vi "DriverStationSendData.vi"   [LabVIEW 2023]
doc: "This VI continously sends data from the robot to the FRC 4265 Dashboard, the joysticks, and the FIRST Driver Station. Data are only sent to the network tables when values change. Detailed sensor data are only sent when the user is currently viewing the Tune tab on the FRC 4265 Dashboard."
uses:
  <vilib>/Rock Robotics/WPI/DriverStation/WPI_DriverStationAllianceInfo.ctl
  0776bb0e-5b58-4af6-957d-bc8a00d122f2.vi
  c0b3d222-824d-4eea-b194-4551ccfede72.vi
  8db4f2bd-6a8b-4c46-90ec-c7212a8cd13c.vi
  7bef9c9e-0ebd-49c4-875e-b1a7c8331b9c.vi
  25034f12-7a14-4040-b0c6-1082a0a618fc.vi
  de71cbf9-497c-4b6e-9325-f91bd1a1ea26.vi
  fe406e7d-1768-469c-a538-67ef48fe7f0a.vi
  b740731d-63e7-4115-93ae-b3fbc4be728c.vi
  770be32f-1451-480f-be59-c95d907125ff.vi
  9b798e4d-9237-4864-9935-e997a6382231.vi
  bf36f1cc-a3b1-4189-9382-aff2debcdd91.vi
  09cab74e-98ba-4de8-92cd-b77291f0cae9.vi
  e0f98f21-d526-4ef5-b75c-6f3c78a33603.vi
  36759aca-d9c6-44a3-918a-9a0e895c718f.vi
  d2dc3f3f-39b5-4c17-a933-05bbedc8d5d9.vi
  47e8091e-0604-4560-b6ee-932fcc40f94c.vi
  040c557e-2b24-4d13-8fef-d98c711cf45f.vi
  89115614-314f-44eb-b4c5-fafba5d31cd4.vi
  9f98788f-6f1b-4a83-a100-7d872b9f460c.vi
  d5b4d43d-cd94-4278-ad04-5030dc28ac17.vi
  c90139ce-4630-4044-962b-b9323bb651b8.vi
  85014151-be37-4cbe-9458-644b8a18b20e.vi
  8274615e-b3b9-4435-b2de-484384c0ad12.vi
  e1fb6d49-71d8-4856-b92a-968cf29c63e6.vi
  9baabde0-90b0-49bc-8c7c-ecb50ab3c219.vi
  7c9ec5b3-0cab-420b-b9c6-0eeed636b797.vi
  a8a67854-f7a1-4059-85f2-a1af3b07aa69.vi
  f0e3ca73-5587-4f60-abb3-83c549356a0b.vi
  135be689-108c-4a89-9837-55c31bad5bbe.vi
  90b8ffb3-02b0-4f37-8578-c415475fcf1f.vi
  26471c2c-aca7-4047-a7cd-e40da11d04c1.vi
  0c9c2ce5-4f8f-4d2f-a61f-dde9fdddd21a.vi
  948ebb5e-1fee-45f5-b788-843df8d92f11.vi
  07cec073-88f4-4f05-94a3-d05e12405c4e.vi
  c10cd8a7-bdb7-4c92-ac5c-00af4ab7dc85.vi
  ce82ba1c-dcc2-498f-8d23-146b12230de2.vi
  cbbdf295-aa1d-4db8-8566-cac5820e4458.vi
  52d993e2-6fbc-4ee4-b085-b3f80a4c3067.vi
  5ccc8aa6-325d-4660-b060-52e30b1d582a.vi
  296afef1-bc02-48ee-92b6-09523bb21575.vi
  811948b9-57e2-4f47-a6f6-f2932d14082f.vi
  5739ca73-a30d-4c92-9c50-72d6edc45fc4.vi
  0620df73-5841-450f-a219-dd10bb38cbc0.vi
  fb087c59-fbb1-4979-ba7d-d29f083bcd8a.vi
  94826c24-d30e-4eee-b4d4-6d626a9b9fe7.vi
  fa7611ee-6daf-4341-84ec-bae2216748b8.vi
  75656f7d-003f-4895-8150-fd75ccee7ba7.vi
  2a5192f0-5560-467f-8dc7-b3093601f5e6.vi
  41cc3bc6-bbb3-49f6-8be0-59cefde1612f.vi
  f5eb47e9-f0d5-4358-ba2d-5c1ea061b043.vi
  7ab91d4b-7be3-4017-93bd-af9165b60b99.vi
  f2a1d575-33e9-46b9-ab25-b575ffc27caf.vi
  2130d5a6-5db2-43ac-bd1b-a97f99664b9f.vi
  375a6e8a-27f7-4291-b992-01fa32110d43.vi
  cffa72e0-3c7a-4932-a37a-7040beb2a623.vi
  ec159192-b170-40c4-82c6-c3d920d678b2.vi
  f6387c7a-a3bd-4a9d-91dd-fe2f33c833ae.vi
  03661406-2ba7-4cad-bba1-149348653281.vi
  d97fc881-b6e7-47be-8bf3-d72bdee58bbc.vi
  29b9fc74-ab20-4616-a405-8bf0304d7e4e.vi
  d8771982-752a-4faa-9266-2bef2163cf3a.vi
  7b6a1411-5027-49fa-871d-ec9f81e31f95.vi
  20dd8ad3-6bbc-4cac-b559-7f798e2b6680.vi
  5e95d400-1295-40c5-af46-ec5444c3a2ff.vi
  d5b53c9f-0752-48c4-83e9-94c6e20357af.vi
  a2a431f6-075f-4920-bddd-4a0a2690fbc3.vi
  63edfc8b-2713-4fb9-bbf0-712b13f7ed91.vi
  5dc304d7-e71b-4cd2-8d9d-954937278b50.vi
  e1c3efee-a4b9-4741-b362-77d4d14dba05.vi
  c227876e-c49d-4561-a8c1-0ac62d9f5df0.vi
  e617f737-58a4-4889-9924-01a8da667f92.vi
  a9076398-35a2-42a7-b542-3dd64d126b59.vi
  44842b00-b9c8-4b1f-a6e0-fc22f00ef89a.vi
  8db4f2bd-6a8b-4c46-90ec-c7212a8cd13c.vi/77c742ae-e671-49bb-a825-a6e8cebc9f63.vi
  7bef9c9e-0ebd-49c4-875e-b1a7c8331b9c.vi/77c742ae-e671-49bb-a825-a6e8cebc9f63.vi
  25034f12-7a14-4040-b0c6-1082a0a618fc.vi/77c742ae-e671-49bb-a825-a6e8cebc9f63.vi
  de71cbf9-497c-4b6e-9325-f91bd1a1ea26.vi/77c742ae-e671-49bb-a825-a6e8cebc9f63.vi
  fe406e7d-1768-469c-a538-67ef48fe7f0a.vi/77c742ae-e671-49bb-a825-a6e8cebc9f63.vi
  b740731d-63e7-4115-93ae-b3fbc4be728c.vi/77c742ae-e671-49bb-a825-a6e8cebc9f63.vi
  770be32f-1451-480f-be59-c95d907125ff.vi/77c742ae-e671-49bb-a825-a6e8cebc9f63.vi
  9b798e4d-9237-4864-9935-e997a6382231.vi/77c742ae-e671-49bb-a825-a6e8cebc9f63.vi
  bf36f1cc-a3b1-4189-9382-aff2debcdd91.vi/77c742ae-e671-49bb-a825-a6e8cebc9f63.vi
  09cab74e-98ba-4de8-92cd-b77291f0cae9.vi/77c742ae-e671-49bb-a825-a6e8cebc9f63.vi
  e0f98f21-d526-4ef5-b75c-6f3c78a33603.vi/77c742ae-e671-49bb-a825-a6e8cebc9f63.vi
  36759aca-d9c6-44a3-918a-9a0e895c718f.vi/77c742ae-e671-49bb-a825-a6e8cebc9f63.vi
  d2dc3f3f-39b5-4c17-a933-05bbedc8d5d9.vi/77c742ae-e671-49bb-a825-a6e8cebc9f63.vi
  47e8091e-0604-4560-b6ee-932fcc40f94c.vi/77c742ae-e671-49bb-a825-a6e8cebc9f63.vi
  040c557e-2b24-4d13-8fef-d98c711cf45f.vi/77c742ae-e671-49bb-a825-a6e8cebc9f63.vi
  89115614-314f-44eb-b4c5-fafba5d31cd4.vi/77c742ae-e671-49bb-a825-a6e8cebc9f63.vi
  9f98788f-6f1b-4a83-a100-7d872b9f460c.vi/77c742ae-e671-49bb-a825-a6e8cebc9f63.vi
  d5b4d43d-cd94-4278-ad04-5030dc28ac17.vi/77c742ae-e671-49bb-a825-a6e8cebc9f63.vi
  c90139ce-4630-4044-962b-b9323bb651b8.vi/77c742ae-e671-49bb-a825-a6e8cebc9f63.vi
  85014151-be37-4cbe-9458-644b8a18b20e.vi/77c742ae-e671-49bb-a825-a6e8cebc9f63.vi
  8274615e-b3b9-4435-b2de-484384c0ad12.vi/77c742ae-e671-49bb-a825-a6e8cebc9f63.vi
  e1fb6d49-71d8-4856-b92a-968cf29c63e6.vi/77c742ae-e671-49bb-a825-a6e8cebc9f63.vi
  9baabde0-90b0-49bc-8c7c-ecb50ab3c219.vi/77c742ae-e671-49bb-a825-a6e8cebc9f63.vi
  7c9ec5b3-0cab-420b-b9c6-0eeed636b797.vi/77c742ae-e671-49bb-a825-a6e8cebc9f63.vi
  a8a67854-f7a1-4059-85f2-a1af3b07aa69.vi/77c742ae-e671-49bb-a825-a6e8cebc9f63.vi
  f0e3ca73-5587-4f60-abb3-83c549356a0b.vi/77c742ae-e671-49bb-a825-a6e8cebc9f63.vi
  135be689-108c-4a89-9837-55c31bad5bbe.vi/77c742ae-e671-49bb-a825-a6e8cebc9f63.vi
  90b8ffb3-02b0-4f37-8578-c415475fcf1f.vi/77c742ae-e671-49bb-a825-a6e8cebc9f63.vi
  26471c2c-aca7-4047-a7cd-e40da11d04c1.vi/77c742ae-e671-49bb-a825-a6e8cebc9f63.vi
  0c9c2ce5-4f8f-4d2f-a61f-dde9fdddd21a.vi/77c742ae-e671-49bb-a825-a6e8cebc9f63.vi
  948ebb5e-1fee-45f5-b788-843df8d92f11.vi/77c742ae-e671-49bb-a825-a6e8cebc9f63.vi
  07cec073-88f4-4f05-94a3-d05e12405c4e.vi/77c742ae-e671-49bb-a825-a6e8cebc9f63.vi
  c10cd8a7-bdb7-4c92-ac5c-00af4ab7dc85.vi/77c742ae-e671-49bb-a825-a6e8cebc9f63.vi
  ce82ba1c-dcc2-498f-8d23-146b12230de2.vi/77c742ae-e671-49bb-a825-a6e8cebc9f63.vi
  cbbdf295-aa1d-4db8-8566-cac5820e4458.vi/77c742ae-e671-49bb-a825-a6e8cebc9f63.vi
  52d993e2-6fbc-4ee4-b085-b3f80a4c3067.vi/77c742ae-e671-49bb-a825-a6e8cebc9f63.vi
  5ccc8aa6-325d-4660-b060-52e30b1d582a.vi/77c742ae-e671-49bb-a825-a6e8cebc9f63.vi
  296afef1-bc02-48ee-92b6-09523bb21575.vi/77c742ae-e671-49bb-a825-a6e8cebc9f63.vi
  811948b9-57e2-4f47-a6f6-f2932d14082f.vi/77c742ae-e671-49bb-a825-a6e8cebc9f63.vi
  5739ca73-a30d-4c92-9c50-72d6edc45fc4.vi/77c742ae-e671-49bb-a825-a6e8cebc9f63.vi
  0620df73-5841-450f-a219-dd10bb38cbc0.vi/77c742ae-e671-49bb-a825-a6e8cebc9f63.vi
  fb087c59-fbb1-4979-ba7d-d29f083bcd8a.vi/77c742ae-e671-49bb-a825-a6e8cebc9f63.vi
  94826c24-d30e-4eee-b4d4-6d626a9b9fe7.vi/77c742ae-e671-49bb-a825-a6e8cebc9f63.vi
  fa7611ee-6daf-4341-84ec-bae2216748b8.vi/77c742ae-e671-49bb-a825-a6e8cebc9f63.vi
  75656f7d-003f-4895-8150-fd75ccee7ba7.vi/77c742ae-e671-49bb-a825-a6e8cebc9f63.vi
  2a5192f0-5560-467f-8dc7-b3093601f5e6.vi/77c742ae-e671-49bb-a825-a6e8cebc9f63.vi
  41cc3bc6-bbb3-49f6-8be0-59cefde1612f.vi/77c742ae-e671-49bb-a825-a6e8cebc9f63.vi
  f5eb47e9-f0d5-4358-ba2d-5c1ea061b043.vi/77c742ae-e671-49bb-a825-a6e8cebc9f63.vi
  7ab91d4b-7be3-4017-93bd-af9165b60b99.vi/77c742ae-e671-49bb-a825-a6e8cebc9f63.vi
  f2a1d575-33e9-46b9-ab25-b575ffc27caf.vi/77c742ae-e671-49bb-a825-a6e8cebc9f63.vi
  2130d5a6-5db2-43ac-bd1b-a97f99664b9f.vi/77c742ae-e671-49bb-a825-a6e8cebc9f63.vi
  375a6e8a-27f7-4291-b992-01fa32110d43.vi/77c742ae-e671-49bb-a825-a6e8cebc9f63.vi
  cffa72e0-3c7a-4932-a37a-7040beb2a623.vi/77c742ae-e671-49bb-a825-a6e8cebc9f63.vi
  ec159192-b170-40c4-82c6-c3d920d678b2.vi/77c742ae-e671-49bb-a825-a6e8cebc9f63.vi
  f6387c7a-a3bd-4a9d-91dd-fe2f33c833ae.vi/77c742ae-e671-49bb-a825-a6e8cebc9f63.vi
  03661406-2ba7-4cad-bba1-149348653281.vi/77c742ae-e671-49bb-a825-a6e8cebc9f63.vi
  d97fc881-b6e7-47be-8bf3-d72bdee58bbc.vi/77c742ae-e671-49bb-a825-a6e8cebc9f63.vi
  29b9fc74-ab20-4616-a405-8bf0304d7e4e.vi/77c742ae-e671-49bb-a825-a6e8cebc9f63.vi
  d8771982-752a-4faa-9266-2bef2163cf3a.vi/77c742ae-e671-49bb-a825-a6e8cebc9f63.vi
  7b6a1411-5027-49fa-871d-ec9f81e31f95.vi/77c742ae-e671-49bb-a825-a6e8cebc9f63.vi
  20dd8ad3-6bbc-4cac-b559-7f798e2b6680.vi/77c742ae-e671-49bb-a825-a6e8cebc9f63.vi
  5e95d400-1295-40c5-af46-ec5444c3a2ff.vi/77c742ae-e671-49bb-a825-a6e8cebc9f63.vi
  d5b53c9f-0752-48c4-83e9-94c6e20357af.vi/77c742ae-e671-49bb-a825-a6e8cebc9f63.vi
  a2a431f6-075f-4920-bddd-4a0a2690fbc3.vi/77c742ae-e671-49bb-a825-a6e8cebc9f63.vi
  63edfc8b-2713-4fb9-bbf0-712b13f7ed91.vi/77c742ae-e671-49bb-a825-a6e8cebc9f63.vi
  5dc304d7-e71b-4cd2-8d9d-954937278b50.vi/77c742ae-e671-49bb-a825-a6e8cebc9f63.vi
  e1c3efee-a4b9-4741-b362-77d4d14dba05.vi/77c742ae-e671-49bb-a825-a6e8cebc9f63.vi
  c227876e-c49d-4561-a8c1-0ac62d9f5df0.vi/77c742ae-e671-49bb-a825-a6e8cebc9f63.vi
  e617f737-58a4-4889-9924-01a8da667f92.vi/77c742ae-e671-49bb-a825-a6e8cebc9f63.vi
  a9076398-35a2-42a7-b542-3dd64d126b59.vi/77c742ae-e671-49bb-a825-a6e8cebc9f63.vi
  44842b00-b9c8-4b1f-a6e0-fc22f00ef89a.vi/77c742ae-e671-49bb-a825-a6e8cebc9f63.vi
  GlobalDriverStationData.vi
  <vilib>/Rock Robotics/Network Tables/NT Write Boolean.vi
  GlobalAutonomous.vi
  <vilib>/Rock Robotics/Network Tables/NT Write String Array.vi
  GlobalDrivebase.vi
  <vilib>/Rock Robotics/Network Tables/NT Write Number.vi
  GlobalMiscellaneous.vi
  <vilib>/Rock Robotics/Network Tables/NT Write String.vi
  GlobalPoseAndTargeting.vi
  Timer.vi
  <vilib>/Rock Robotics/Network Tables/NT Write Boolean Array.vi
  GlobalElevator.vi
  GlobalNoteHandling.vi
  GlobalShooter.vi
  <vilib>/Rock Robotics/Network Tables/NT Write Variant.vi
  <vilib>/Rock Robotics/Network Tables/NT Write Numeric Array.vi
  <vilib>/Rock Robotics/Network Tables/NT Write Float Array.vi
  <vilib>/Rock Robotics/Network Tables/NT Write Integer.vi
types:
  T1 = typedef "WPI_DriverStationAllianceInfo.ctl" = enum16{"Red", "Blue", "Invalid"}
  T2 = enum16{"Low Gear", "High Gear", "Transiting", "Unknown", "Force Low Gear"}
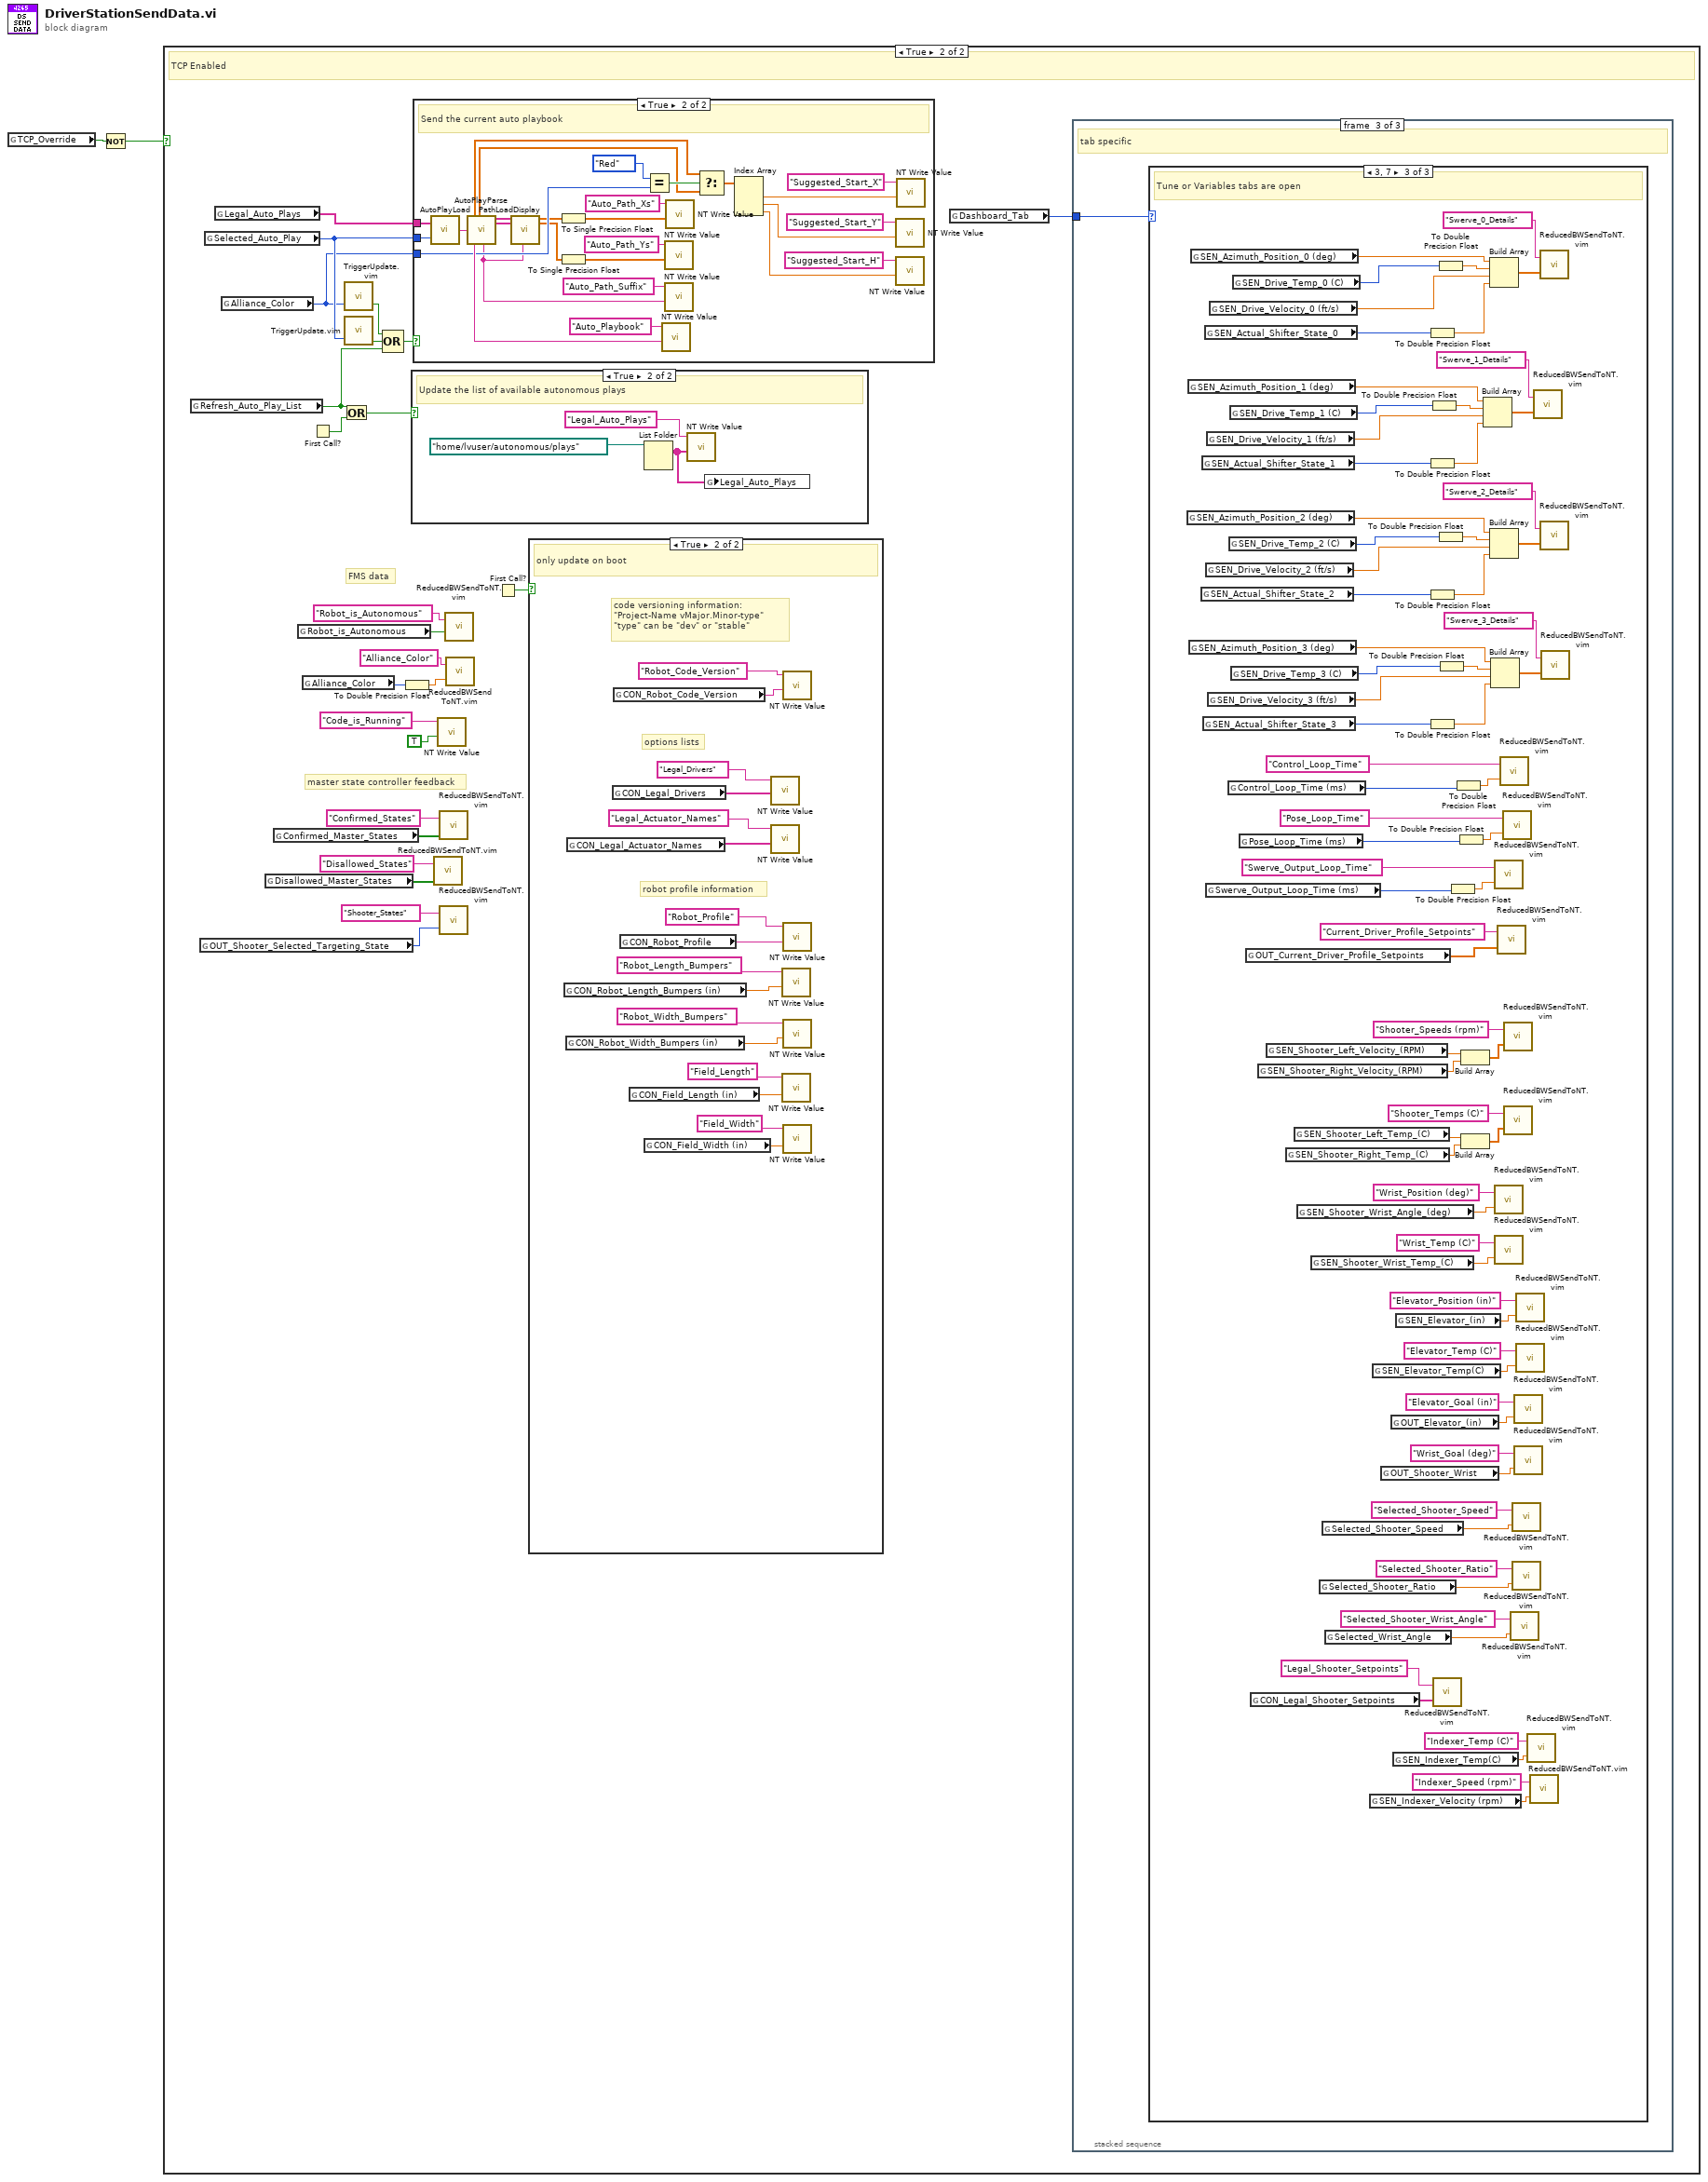
[diagram p0: block diagram]
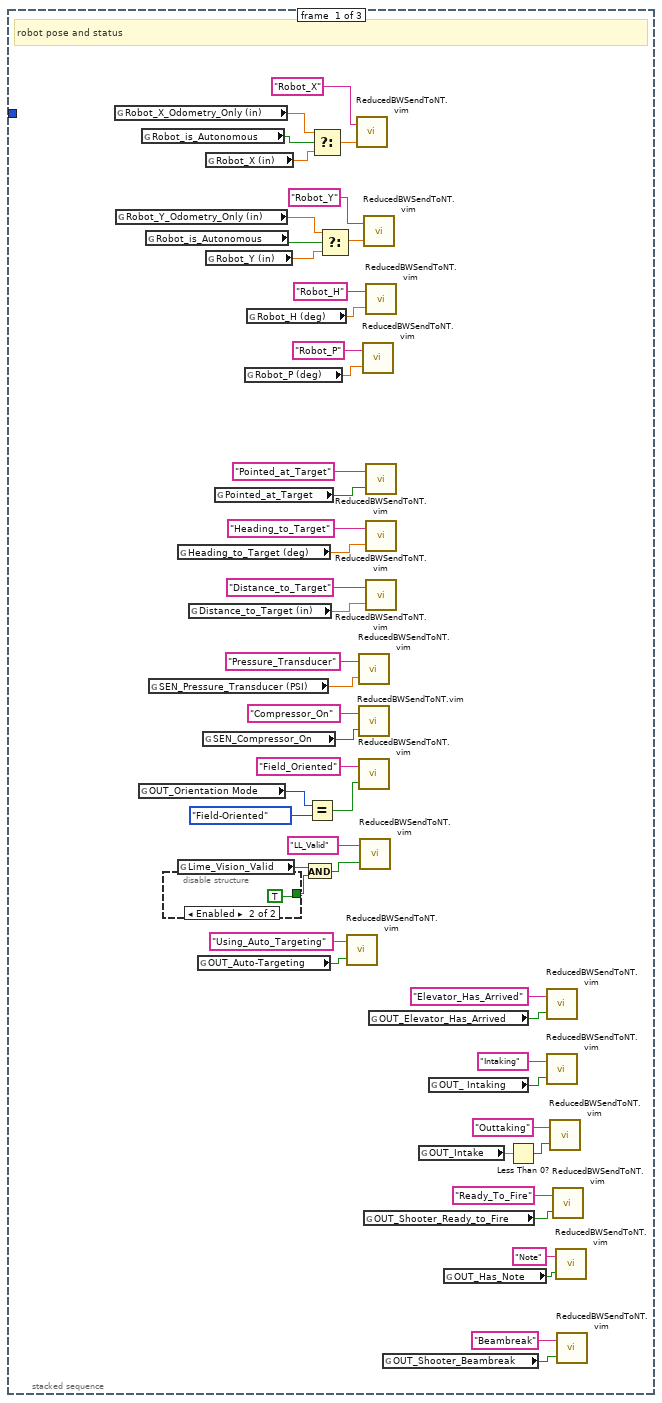
[diagram p3: hidden frame]
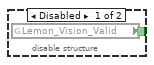
[diagram p4: hidden frame]
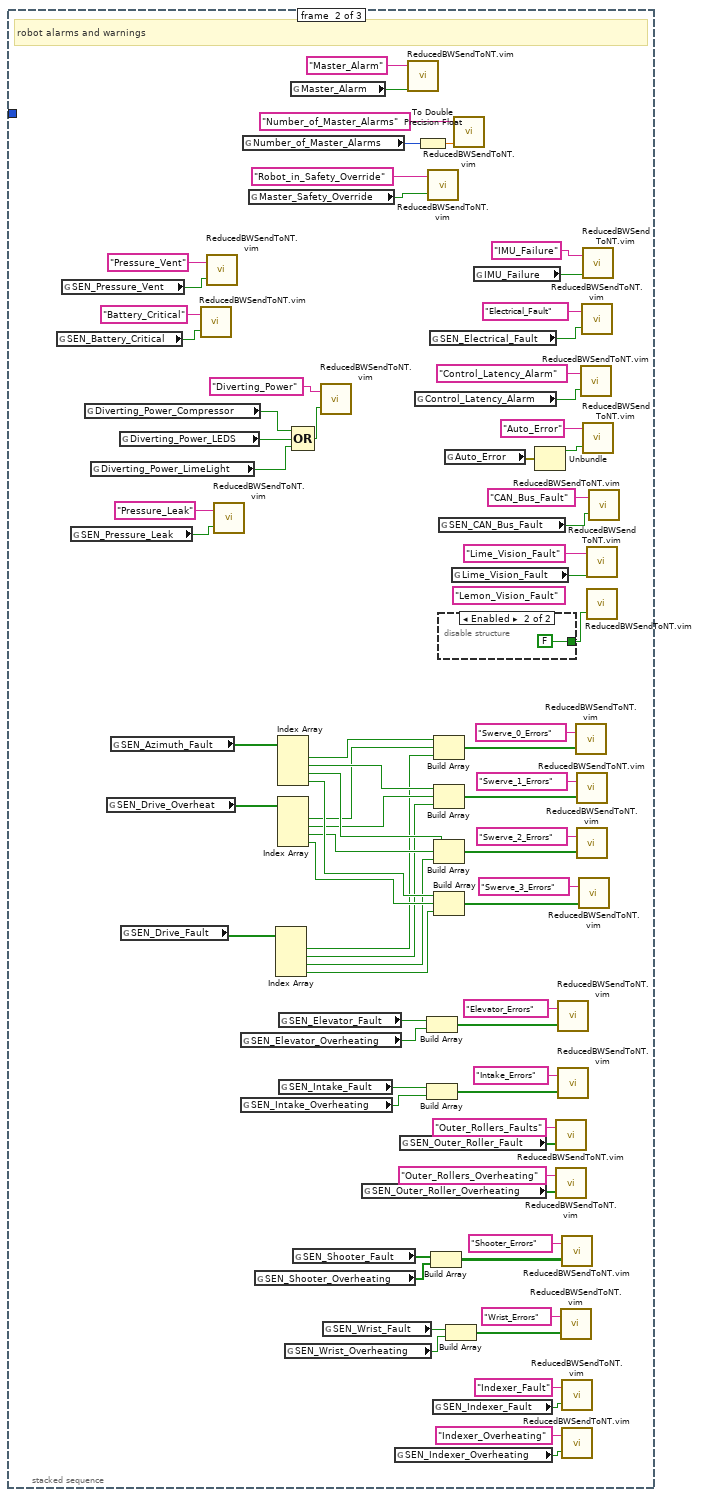
[diagram p5: hidden frame]
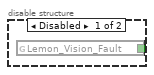
[diagram p6: hidden frame]
diagram:
  n1 = global read "GlobalDriverStationData.vi" "TCP_Override"() -> (w2:bool)
  n2 = Not(x=w2) -> (.not. x?=w1:bool)
  n3 = case shown="True" w1 {
    frame False {
      # "TCP Disabled"
    }
    frame True {
      # "FMS data"
      # "master state controller feedback"
      # "TCP Enabled"
      n4 = global read "GlobalDriverStationData.vi" "Refresh_Auto_Play_List"() -> (w22:bool)
      n5 = global read "GlobalShooter.vi" "OUT_Shooter_Selected_Targeting_State"() -> (w3:enum16{"TACO", "Subwoofer", "Stage"})
      n6 = global read "GlobalDriverStationData.vi" "Selected_Auto_Play"() -> (w9:u16)
      n7 = global read "GlobalAutonomous.vi" "Legal_Auto_Plays"() -> (w10:string[])
      n8 = global read "GlobalDriverStationData.vi" "Alliance_Color"() -> (w7:T1)
      n9 = global read "GlobalMiscellaneous.vi" "Disallowed_Master_States"() -> (w12:bool[])
      n10 = global read "GlobalMiscellaneous.vi" "Confirmed_Master_States"() -> (w14:bool[])
      n11 = global read "GlobalDriverStationData.vi" "Robot_is_Autonomous"() -> (w18:bool)
      n12 = global read "GlobalDriverStationData.vi" "Alliance_Color"() -> (w20:T1)
      n13 = First Call?() -> (First Call?: T/F=w26:bool)
      n14 = Or(x=w22, y=w26) -> (x .or. y?=w25:bool)
      n15 = call "TriggerUpdate.vim"("Trigger"=w7) -> ("Update"=w8:bool)  [unwired: 2 in]
      n16 = call "TriggerUpdate.vim"("Trigger"=w9) -> ("Update"=w24:bool)  [unwired: 2 in]
      n17 = Compound Arithmetic op=OR(w8, w24, w22) -> (w23:bool)
      n18 = To Double Precision Float(number=w20) -> (double precision float=w16:dbl)
      n19 = case shown="True" w25 {
        frame False {
        }
        frame True {
          # "Update the list of available autonomous plays"
          n20 = List Folder(path=path "/home/lvuser/autonomous/plays") -> (filenames=w276:string[])  [unwired: 3 in, 3 out]
          n21 = call-poly <vilib>:"NT Write Value.vi"("value"=w276, "name"="Legal_Auto_Plays" ("Name")) -> ()  [unwired: 9 in, 1 out]
          n22 = global write "GlobalAutonomous.vi" "Legal_Auto_Plays"(w276) -> ()
        }
      }
      n23 = case shown="True" w23 {
        tunnel: w9 -> [_ w273]
        tunnel: w10 -> [_ w272]
        tunnel: w7 -> [_ w268]
        frame False {
        }
        frame True {
          # "Send the current auto playbook"
          n24 = call "AutoPlayLoad.vi"("Selected Auto Play"=w273, "Available Auto Plays"=w272) -> ("Loaded Auto Play"=w274:string)
          n25 = call "AutoPlayParse.vi"("Loaded Auto Play"=w274) -> ("Suggested Start Red"=w266:dbl[], "Full Auto Play Text"=w271:string, "Suggested Start Blue"=w265:dbl[], "Autonomous Path Suffix"=w255:string, "Drive Command Strings"=w257:string[], "Drive Parameter Strings"=w256:string[])  [unwired: 10 in, 3 out]
          n26 = call "PathLoadDisplay.vi"("Drive Command Strings"=w257, "Drive Parameter Strings"=w256, "Autonomous Path Suffix"=w255) -> ("Path X Coordinates (in)"=w253:dbl[], "Path Y Coordinates (in)"=w251:dbl[])  [unwired: 15 in]
          n27 = To Single Precision Float(number=w253) -> (single precision float=w250:sgl[])
          n28 = To Single Precision Float(number=w251) -> (single precision float=w249:sgl[])
          n29 = Equal?(x=WPI_DriverStationAllianceInfo."Red", y=w268) -> (x = y?=w269:bool)
          n30 = call-poly <vilib>:"NT Write Value.vi"("value"=w271, "name"="Auto_Playbook" ("Name")) -> ()  [unwired: 9 in, 1 out]
          n31 = call-poly <vilib>:"NT Write Value.vi"("value"=w249, "name"="Auto_Path_Ys" ("Name")) -> ()  [unwired: 9 in, 1 out]
          n32 = call-poly <vilib>:"NT Write Value.vi"("value"=w255, "name"="Auto_Path_Suffix" ("Name")) -> ()  [unwired: 9 in, 1 out]
          n33 = call-poly <vilib>:"NT Write Value.vi"("value"=w250, "name"="Auto_Path_Xs" ("Name")) -> ()  [unwired: 9 in, 1 out]
          n34 = Select(t=w266, s=w269, f=w265) -> (s? t:f=w264:dbl[])
          n35 = Index Array(array=w264) -> (element #1=w260:dbl, element #2=w259:dbl, element #3=w258:dbl)  [unwired: 3 in]
          n36 = call-poly <vilib>:"NT Write Value.vi"("value"=w259, "name"="Suggested_Start_Y" ("Name")) -> ()  [unwired: 9 in, 1 out]
          n37 = call-poly <vilib>:"NT Write Value.vi"("value"=w258, "name"="Suggested_Start_H" ("Name")) -> ()  [unwired: 9 in, 1 out]
          n38 = call-poly <vilib>:"NT Write Value.vi"("value"=w260, "name"="Suggested_Start_X" ("Name")) -> ()  [unwired: 9 in, 1 out]
        }
      }
      n39 = call "ReducedBWSendToNT.vim"("Value In"=w12, "NT Name"="Disallowed_States" ("Name")) -> ()  [unwired: 1 out]
      n40 = call-poly <vilib>:"NT Write Value.vi"("value"=TRUE, "name"="Code_is_Running" ("NT Name")) -> ()  [unwired: 9 in, 1 out]
      n41 = call "ReducedBWSendToNT.vim"("Value In"=w14, "NT Name"="Confirmed_States" ("Name")) -> ()  [unwired: 1 out]
      n42 = call "ReducedBWSendToNT.vim"("Value In"=w3, "NT Name"="Shooter_States" ("Name")) -> ()  [unwired: 1 out]
      n43 = call "ReducedBWSendToNT.vim"("Value In"=w18, "NT Name"="Robot_is_Autonomous") -> ()  [unwired: 1 out]
      n44 = call "ReducedBWSendToNT.vim"("Value In"=w16, "NT Name"="Alliance_Color") -> ()  [unwired: 1 out]
      n45 = First Call?() -> (First Call?: T/F=w21:bool)
      n46 = case shown="True" w21 {
        frame False {
        }
        frame True {
          # "robot profile information"
          # "options lists"
          # "code versioning information:\n\"Project-Name vMajor.Minor-type\"\n\"type\" can be \"dev\" or \"stable\""
          # "only update on boot"
          n47 = global read "GlobalDrivebase.vi" "CON_Robot_Length_Bumpers (in)"() -> (w242:dbl)
          n48 = global read "GlobalDrivebase.vi" "CON_Robot_Width_Bumpers (in)"() -> (w241:dbl)
          n49 = global read "GlobalMiscellaneous.vi" "CON_Legal_Actuator_Names"() -> (w239:string[])
          n50 = global read "GlobalDrivebase.vi" "CON_Legal_Drivers"() -> (w240:string[])
          n51 = global read "GlobalMiscellaneous.vi" "CON_Robot_Code_Version"() -> (w237:string)
          n52 = global read "GlobalMiscellaneous.vi" "CON_Robot_Profile"() -> (w238:string)
          n53 = global read "GlobalPoseAndTargeting.vi" "CON_Field_Length (in)"() -> (w236:dbl)
          n54 = global read "GlobalPoseAndTargeting.vi" "CON_Field_Width (in)"() -> (w233:dbl)
          n55 = call-poly <vilib>:"NT Write Value.vi"("value"=w240, "name"="Legal_Drivers" ("Name")) -> ()  [unwired: 9 in, 1 out]
          n56 = call-poly <vilib>:"NT Write Value.vi"("value"=w239, "name"="Legal_Actuator_Names" ("Name")) -> ()  [unwired: 9 in, 1 out]
          n57 = call-poly <vilib>:"NT Write Value.vi"("value"=w242, "name"="Robot_Length_Bumpers" ("Name")) -> ()  [unwired: 9 in, 1 out]
          n58 = call-poly <vilib>:"NT Write Value.vi"("value"=w236, "name"="Field_Length" ("Name")) -> ()  [unwired: 9 in, 1 out]
          n59 = call-poly <vilib>:"NT Write Value.vi"("value"=w237, "name"="Robot_Code_Version" ("Name")) -> ()  [unwired: 9 in, 1 out]
          n60 = call-poly <vilib>:"NT Write Value.vi"("value"=w238, "name"="Robot_Profile" ("Name")) -> ()  [unwired: 9 in, 1 out]
          n61 = call-poly <vilib>:"NT Write Value.vi"("value"=w241, "name"="Robot_Width_Bumpers" ("Name")) -> ()  [unwired: 9 in, 1 out]
          n62 = call-poly <vilib>:"NT Write Value.vi"("value"=w233, "name"="Field_Width" ("Name")) -> ()  [unwired: 9 in, 1 out]
        }
      }
      n63 = global read "GlobalDriverStationData.vi" "Dashboard_Tab"() -> (w11:i8)
      n64 = stacked-sequence {
        tunnel: w11 -> [_ _ w157]
        frame #0 {
          # "robot pose and status"
          n65 = global read "GlobalPoseAndTargeting.vi" "Robot_X_Odometry_Only (in)"() -> (w68:dbl)
          n66 = global read "GlobalPoseAndTargeting.vi" "Robot_Y_Odometry_Only (in)"() -> (w69:dbl)
          n67 = global read "GlobalDrivebase.vi" "OUT_Orientation Mode"() -> (w55:enum16{"Robot-Oriented", "Field-Oriented"})
          n68 = global read "GlobalDriverStationData.vi" "Robot_is_Autonomous"() -> (w72:bool)
          n69 = global read "GlobalDriverStationData.vi" "Robot_is_Autonomous"() -> (w73:bool)
          n70 = global read "GlobalMiscellaneous.vi" "SEN_Pressure_Transducer (PSI)"() -> (w54:dbl)
          n71 = disable-structure shown="Enabled" {
            disable-tunnel: [w74 TRUE ("Lemon_Vision_Valid")] -> w28
            frame Disabled {
              n72 = global read "GlobalPoseAndTargeting.vi" "Lemon_Vision_Valid"() -> (w74:bool)
            }
            frame Enabled {
            }
          }
          n73 = global read "GlobalPoseAndTargeting.vi" "Heading_to_Target (deg)"() -> (w48:dbl)
          n74 = global read "GlobalPoseAndTargeting.vi" "Lime_Vision_Valid"() -> (w29:bool)
          n75 = global read "GlobalPoseAndTargeting.vi" "Distance_to_Target (in)"() -> (w46:dbl)
          n76 = global read "GlobalDrivebase.vi" "OUT_Auto-Targeting"() -> (w43:bool)
          n77 = global read "GlobalMiscellaneous.vi" "SEN_Compressor_On"() -> (w53:bool)
          n78 = global read "GlobalPoseAndTargeting.vi" "Robot_X (in)"() -> (w66:dbl)
          n79 = global read "GlobalPoseAndTargeting.vi" "Robot_Y (in)"() -> (w67:dbl)
          n80 = global read "GlobalPoseAndTargeting.vi" "Pointed_at_Target"() -> (w50:bool)
          n81 = global read "GlobalPoseAndTargeting.vi" "Robot_P (deg)"() -> (w52:dbl)
          n82 = global read "GlobalPoseAndTargeting.vi" "Robot_H (deg)"() -> (w65:dbl)
          n83 = And(x=w29, y=w28) -> (x .and. y?=w30:bool)
          n84 = Equal?(x=w55, y=enum16{"Robot-Oriented", "Field-Oriented"}."Field-Oriented") -> (x = y?=w61:bool)
          n85 = Select(t=w68, s=w72, f=w66) -> (s? t:f=w70:dbl)
          n86 = Select(t=w69, s=w73, f=w67) -> (s? t:f=w71:dbl)
          n87 = call "ReducedBWSendToNT.vim"("Value In"=w43, "NT Name"="Using_Auto_Targeting" ("Name")) -> ()  [unwired: 1 out]
          n88 = call "ReducedBWSendToNT.vim"("Value In"=w70, "NT Name"="Robot_X" ("Name")) -> ()  [unwired: 1 out]
          n89 = call "ReducedBWSendToNT.vim"("Value In"=w54, "NT Name"="Pressure_Transducer" ("Name")) -> ()  [unwired: 1 out]
          n90 = call "ReducedBWSendToNT.vim"("Value In"=w53, "NT Name"="Compressor_On" ("Name")) -> ()  [unwired: 1 out]
          n91 = call "ReducedBWSendToNT.vim"("Value In"=w61, "NT Name"="Field_Oriented" ("Name")) -> ()  [unwired: 1 out]
          n92 = call "ReducedBWSendToNT.vim"("Value In"=w30, "NT Name"="LL_Valid" ("Name")) -> ()  [unwired: 1 out]
          n93 = call "ReducedBWSendToNT.vim"("Value In"=w52, "NT Name"="Robot_P" ("Name")) -> ()  [unwired: 1 out]
          n94 = call "ReducedBWSendToNT.vim"("Value In"=w71, "NT Name"="Robot_Y" ("Name")) -> ()  [unwired: 1 out]
          n95 = global read "GlobalShooter.vi" "OUT_Shooter_Ready_to_Fire"() -> (w34:bool)
          n96 = call "ReducedBWSendToNT.vim"("Value In"=w65, "NT Name"="Robot_H" ("Name")) -> ()  [unwired: 1 out]
          n97 = call "ReducedBWSendToNT.vim"("Value In"=w50, "NT Name"="Pointed_at_Target" ("Name")) -> ()  [unwired: 1 out]
          n98 = call "ReducedBWSendToNT.vim"("Value In"=w48, "NT Name"="Heading_to_Target" ("Name")) -> ()  [unwired: 1 out]
          n99 = call "ReducedBWSendToNT.vim"("Value In"=w46, "NT Name"="Distance_to_Target" ("Name")) -> ()  [unwired: 1 out]
          n100 = global read "GlobalElevator.vi" "OUT_Elevator_Has_Arrived"() -> (w42:bool)
          n101 = global read "GlobalNoteHandling.vi" "OUT_Shooter_Beambreak"() -> (w31:bool)
          n102 = global read "GlobalNoteHandling.vi" "OUT_Intake"() -> (w37:dbl)
          n103 = global read "GlobalNoteHandling.vi" "OUT_ Intaking"() -> (w38:bool)
          n104 = global read "GlobalNoteHandling.vi" "OUT_Has_Note"() -> (w27:bool)
          n105 = Less Than 0?(x=w37) -> (x < 0?=w36:bool)
          n106 = call "ReducedBWSendToNT.vim"("Value In"=w42, "NT Name"="Elevator_Has_Arrived") -> ()  [unwired: 1 out]
          n107 = call "ReducedBWSendToNT.vim"("Value In"=w38, "NT Name"="Intaking") -> ()  [unwired: 1 out]
          n108 = call "ReducedBWSendToNT.vim"("Value In"=w36, "NT Name"="Outtaking") -> ()  [unwired: 1 out]
          n109 = call "ReducedBWSendToNT.vim"("Value In"=w34, "NT Name"="Ready_To_Fire") -> ()  [unwired: 1 out]
          n110 = call "ReducedBWSendToNT.vim"("Value In"=w27, "NT Name"="Note") -> ()  [unwired: 1 out]
          n111 = call "ReducedBWSendToNT.vim"("Value In"=w31, "NT Name"="Beambreak") -> ()  [unwired: 1 out]
        }
        frame #1 {
          (unwired) "Lemon_Vision_Fault" ("Name")
          # "robot alarms and warnings"
          n112 = global read "GlobalMiscellaneous.vi" "SEN_Battery_Critical"() -> (w110:bool)
          n113 = global read "GlobalMiscellaneous.vi" "SEN_Pressure_Vent"() -> (w111:bool)
          n114 = global read "GlobalMiscellaneous.vi" "SEN_Pressure_Leak"() -> (w107:bool)
          n115 = global read "GlobalMiscellaneous.vi" "Diverting_Power_Compressor"() -> (w146:bool)
          n116 = global read "GlobalMiscellaneous.vi" "Diverting_Power_LimeLight"() -> (w148:bool)
          n117 = global read "GlobalDrivebase.vi" "SEN_Drive_Overheat"() -> (w112:bool[])
          n118 = global read "GlobalDrivebase.vi" "SEN_Azimuth_Fault"() -> (w113:bool[])
          n119 = global read "GlobalMiscellaneous.vi" "Diverting_Power_LEDS"() -> (w147:bool)
          n120 = global read "GlobalDrivebase.vi" "SEN_Drive_Fault"() -> (w105:bool[])
          n121 = call "ReducedBWSendToNT.vim"("Value In"=w110, "NT Name"="Battery_Critical" ("Name")) -> ()  [unwired: 1 out]
          n122 = call "ReducedBWSendToNT.vim"("Value In"=w111, "NT Name"="Pressure_Vent" ("Name")) -> ()  [unwired: 1 out]
          n123 = call "ReducedBWSendToNT.vim"("Value In"=w107, "NT Name"="Pressure_Leak" ("Name")) -> ()  [unwired: 1 out]
          n124 = global read "GlobalElevator.vi" "SEN_Elevator_Overheating"() -> (w98:bool)
          n125 = global read "GlobalNoteHandling.vi" "SEN_Intake_Overheating"() -> (w91:bool)
          n126 = global read "GlobalMiscellaneous.vi" "Number_of_Master_Alarms"() -> (w153:i32)
          n127 = global read "GlobalDriverStationData.vi" "Master_Safety_Override"() -> (w149:bool)
          n128 = global read "GlobalShooter.vi" "SEN_Shooter_Overheating"() -> (w89:bool[])
          n129 = Index Array(array=w105) -> (element #1=w104:bool, element #2=w103:bool, element #3=w102:bool, element #4=w101:bool)  [unwired: 4 in]
          n130 = Index Array(array=w113) -> (element #1=w120:bool, element #2=w122:bool, element #3=w124:bool, element #4=w126:bool)  [unwired: 4 in]
          n131 = Index Array(array=w112) -> (element #1=w121:bool, element #2=w123:bool, element #3=w125:bool, element #4=w127:bool)  [unwired: 4 in]
          n132 = global read "GlobalElevator.vi" "SEN_Elevator_Fault"() -> (w97:bool)
          n133 = global read "GlobalNoteHandling.vi" "SEN_Intake_Fault"() -> (w92:bool)
          n134 = global read "GlobalShooter.vi" "SEN_Wrist_Overheating"() -> (w84:bool)
          n135 = global read "GlobalMiscellaneous.vi" "Master_Alarm"() -> (w152:bool)
          n136 = Compound Arithmetic op=OR(w146, w147, w148) -> (w145:bool)
          n137 = global read "GlobalShooter.vi" "SEN_Shooter_Fault"() -> (w90:bool[])
          n138 = call "ReducedBWSendToNT.vim"("Value In"=w145, "NT Name"="Diverting_Power" ("Name")) -> ()  [unwired: 1 out]
          n139 = global read "GlobalShooter.vi" "SEN_Wrist_Fault"() -> (w83:bool)
          n140 = global read "GlobalNoteHandling.vi" "SEN_Outer_Roller_Overheating"() -> (w85:bool[])
          n141 = global read "GlobalNoteHandling.vi" "SEN_Indexer_Overheating"() -> (w79:bool)
          n142 = global read "GlobalNoteHandling.vi" "SEN_Outer_Roller_Fault"() -> (w86:bool[])
          n143 = call "ReducedBWSendToNT.vim"("Value In"=w152, "NT Name"="Master_Alarm" ("Name")) -> ()  [unwired: 1 out]
          n144 = global read "GlobalMiscellaneous.vi" "Control_Latency_Alarm"() -> (w108:bool)
          n145 = To Double Precision Float(number=w153) -> (double precision float=w154:dbl)
          n146 = Build Array(w97, w98) -> (w99:bool[])
          n147 = Build Array(w92, w91) -> (w96:bool[])
          n148 = call "ReducedBWSendToNT.vim"("Value In"=w149, "NT Name"="Robot_in_Safety_Override" ("Name")) -> ()  [unwired: 1 out]
          n149 = global read "GlobalMiscellaneous.vi" "SEN_Electrical_Fault"() -> (w109:bool)
          n150 = Build Array(w90, w89) -> (w93:bool[][])
          n151 = global read "GlobalNoteHandling.vi" "SEN_Indexer_Fault"() -> (w78:bool)
          n152 = Build Array(w120, w121, w104) -> (w128:bool[])
          n153 = Build Array(w122, w123, w103) -> (w129:bool[])
          n154 = Build Array(w124, w125, w102) -> (w130:bool[])
          n155 = Build Array(w126, w127, w101) -> (w131:bool[])
          n156 = global read "GlobalMiscellaneous.vi" "SEN_CAN_Bus_Fault"() -> (w106:bool)
          n157 = disable-structure shown="Enabled" {
            disable-tunnel: [w155 FALSE ("Lemon_Vision_Fault")] -> w80
            frame Disabled {
              n158 = global read "GlobalPoseAndTargeting.vi" "Lemon_Vision_Fault"() -> (w155:bool)
            }
            frame Enabled {
            }
          }
          n159 = global read "GlobalAutonomous.vi" "Auto_Error"() -> (w142:errorcluster)
          n160 = Build Array(w83, w84) -> (w82:bool[])
          n161 = global read "GlobalPoseAndTargeting.vi" "Lime_Vision_Fault"() -> (w132:bool)
          n162 = call "ReducedBWSendToNT.vim"("Value In"=w154, "NT Name"="Number_of_Master_Alarms" ("Name")) -> ()  [unwired: 1 out]
          n163 = global read "GlobalPoseAndTargeting.vi" "IMU_Failure"() -> (w144:bool)
          n164 = Unbundle(w142) -> ("status"=w143:bool)  [unwired: 2 out]
          n165 = call "ReducedBWSendToNT.vim"("Value In"=w86, "NT Name"="Outer_Rollers_Faults") -> ()  [unwired: 1 out]
          n166 = call "ReducedBWSendToNT.vim"("Value In"=w85, "NT Name"="Outer_Rollers_Overheating") -> ()  [unwired: 1 out]
          n167 = call "ReducedBWSendToNT.vim"("Value In"=w99, "NT Name"="Elevator_Errors") -> ()  [unwired: 1 out]
          n168 = call "ReducedBWSendToNT.vim"("Value In"=w96, "NT Name"="Intake_Errors") -> ()  [unwired: 1 out]
          n169 = call "ReducedBWSendToNT.vim"("Value In"=w82, "NT Name"="Wrist_Errors") -> ()  [unwired: 1 out]
          n170 = call "ReducedBWSendToNT.vim"("Value In"=w93, "NT Name"="Shooter_Errors") -> ()  [unwired: 1 out]
          n171 = call "ReducedBWSendToNT.vim"("Value In"=w78, "NT Name"="Indexer_Fault") -> ()  [unwired: 1 out]
          n172 = call "ReducedBWSendToNT.vim"("Value In"=w79, "NT Name"="Indexer_Overheating") -> ()  [unwired: 1 out]
          n173 = call "ReducedBWSendToNT.vim"("Value In"=w128, "NT Name"="Swerve_0_Errors") -> ()  [unwired: 1 out]
          n174 = call "ReducedBWSendToNT.vim"("Value In"=w129, "NT Name"="Swerve_1_Errors") -> ()  [unwired: 1 out]
          n175 = call "ReducedBWSendToNT.vim"("Value In"=w130, "NT Name"="Swerve_2_Errors") -> ()  [unwired: 1 out]
          n176 = call "ReducedBWSendToNT.vim"("Value In"=w131, "NT Name"="Swerve_3_Errors") -> ()  [unwired: 1 out]
          n177 = call "ReducedBWSendToNT.vim"("Value In"=w108, "NT Name"="Control_Latency_Alarm" ("Name")) -> ()  [unwired: 1 out]
          n178 = call "ReducedBWSendToNT.vim"("Value In"=w109, "NT Name"="Electrical_Fault" ("Name")) -> ()  [unwired: 1 out]
          n179 = call "ReducedBWSendToNT.vim"("Value In"=w144, "NT Name"="IMU_Failure" ("Name")) -> ()  [unwired: 1 out]
          n180 = call "ReducedBWSendToNT.vim"("Value In"=w143, "NT Name"="Auto_Error" ("Name")) -> ()  [unwired: 1 out]
          n181 = call "ReducedBWSendToNT.vim"("Value In"=w132, "NT Name"="Lime_Vision_Fault" ("Name")) -> ()  [unwired: 1 out]
          n182 = call "ReducedBWSendToNT.vim"("Value In"=w80) -> ()  [unwired: 1 in, 1 out]
          n183 = call "ReducedBWSendToNT.vim"("Value In"=w106, "NT Name"="CAN_Bus_Fault" ("Name")) -> ()  [unwired: 1 out]
        }
        frame #2 {
          # "tab specific"
          n184 = case shown="3, 7" w157 {
            frame 0, Default {
              # "no tab open"
            }
            frame 1 {
              # "Auto/Setup tab open"
            }
            frame 3, 7 {
              # "Tune or Variables tabs are open"
              n185 = global read "GlobalDrivebase.vi" "SEN_Azimuth_Position_2 (deg)"() -> (w206:dbl)
              n186 = global read "GlobalDrivebase.vi" "SEN_Azimuth_Position_1 (deg)"() -> (w209:dbl)
              n187 = global read "GlobalDrivebase.vi" "SEN_Azimuth_Position_3 (deg)"() -> (w203:dbl)
              n188 = global read "GlobalDrivebase.vi" "SEN_Azimuth_Position_0 (deg)"() -> (w212:dbl)
              n189 = global read "GlobalDrivebase.vi" "SEN_Actual_Shifter_State_2"() -> (w159:T2)
              n190 = global read "GlobalDrivebase.vi" "SEN_Actual_Shifter_State_1"() -> (w160:T2)
              n191 = global read "GlobalDrivebase.vi" "SEN_Actual_Shifter_State_3"() -> (w158:T2)
              n192 = global read "GlobalDrivebase.vi" "SEN_Actual_Shifter_State_0"() -> (w161:T2)
              n193 = global read "GlobalDrivebase.vi" "SEN_Drive_Velocity_2 (ft/s)"() -> (w204:dbl)
              n194 = global read "GlobalMiscellaneous.vi" "Swerve_Output_Loop_Time (ms)"() -> (w196:u32)
              n195 = global read "GlobalDrivebase.vi" "SEN_Drive_Velocity_1 (ft/s)"() -> (w207:dbl)
              n196 = global read "GlobalDrivebase.vi" "SEN_Drive_Velocity_3 (ft/s)"() -> (w201:dbl)
              n197 = global read "GlobalDrivebase.vi" "SEN_Drive_Velocity_0 (ft/s)"() -> (w210:dbl)
              n198 = global read "GlobalMiscellaneous.vi" "Control_Loop_Time (ms)"() -> (w200:u32)
              n199 = global read "GlobalDrivebase.vi" "SEN_Drive_Temp_2 (C)"() -> (w205:u8)
              n200 = global read "GlobalDrivebase.vi" "SEN_Drive_Temp_1 (C)"() -> (w208:u8)
              n201 = global read "GlobalDrivebase.vi" "SEN_Drive_Temp_3 (C)"() -> (w202:u8)
              n202 = global read "GlobalDrivebase.vi" "SEN_Drive_Temp_0 (C)"() -> (w211:u8)
              n203 = global read "GlobalMiscellaneous.vi" "Pose_Loop_Time (ms)"() -> (w199:u32)
              n204 = global read "GlobalDrivebase.vi" "OUT_Current_Driver_Profile_Setpoints"() -> (w213:dbl[])
              n205 = global read "GlobalShooter.vi" "CON_Legal_Shooter_Setpoints"() -> (w166:string[])
              n206 = global read "GlobalShooter.vi" "SEN_Shooter_Right_Velocity_(RPM)"() -> (w194:dbl)
              n207 = global read "GlobalShooter.vi" "SEN_Shooter_Left_Velocity_(RPM)"() -> (w195:dbl)
              n208 = global read "GlobalShooter.vi" "SEN_Shooter_Right_Temp_(C)"() -> (w191:dbl)
              n209 = global read "GlobalShooter.vi" "SEN_Shooter_Left_Temp_(C)"() -> (w190:dbl)
              n210 = global read "GlobalShooter.vi" "SEN_Shooter_Wrist_Angle_(deg)"() -> (w189:dbl)
              n211 = global read "GlobalShooter.vi" "SEN_Shooter_Wrist_Temp_(C)"() -> (w188:dbl)
              n212 = global read "GlobalShooter.vi" "Selected_Shooter_Ratio"() -> (w170:dbl)
              n213 = global read "GlobalShooter.vi" "Selected_Shooter_Speed"() -> (w173:dbl)
              n214 = global read "GlobalShooter.vi" "Selected_Wrist_Angle"() -> (w169:dbl)
              n215 = global read "GlobalNoteHandling.vi" "SEN_Indexer_Velocity (rpm)"() -> (w162:dbl)
              n216 = global read "GlobalElevator.vi" "SEN_Elevator_Temp(C)"() -> (w180:dbl)
              n217 = global read "GlobalShooter.vi" "OUT_Shooter_Wrist"() -> (w176:dbl)
              n218 = global read "GlobalElevator.vi" "OUT_Elevator_(in)"() -> (w179:dbl)
              n219 = global read "GlobalNoteHandling.vi" "SEN_Indexer_Temp(C)"() -> (w165:dbl)
              n220 = global read "GlobalElevator.vi" "SEN_Elevator_(in)"() -> (w181:dbl)
              n221 = To Double Precision Float(number=w161) -> (double precision float=w175:dbl)
              n222 = To Double Precision Float(number=w160) -> (double precision float=w223:dbl)
              n223 = To Double Precision Float(number=w159) -> (double precision float=w174:dbl)
              n224 = To Double Precision Float(number=w158) -> (double precision float=w216:dbl)
              n225 = To Double Precision Float(number=w208) -> (double precision float=w224:dbl)
              n226 = call "ReducedBWSendToNT.vim"("Value In"=w166, "NT Name"="Legal_Shooter_Setpoints" ("Name")) -> ()  [unwired: 1 out]
              n227 = To Double Precision Float(number=w211) -> (double precision float=w227:dbl)
              n228 = To Double Precision Float(number=w205) -> (double precision float=w220:dbl)
              n229 = To Double Precision Float(number=w202) -> (double precision float=w217:dbl)
              n230 = To Double Precision Float(number=w196) -> (double precision float=w197:dbl)
              n231 = To Double Precision Float(number=w200) -> (double precision float=w231:dbl)
              n232 = To Double Precision Float(number=w199) -> (double precision float=w229:dbl)
              n233 = Build Array(w195, w194) -> (w193:dbl[])
              n234 = Build Array(w190, w191) -> (w192:dbl[])
              n235 = Build Array(w209, w224, w207, w223) -> (w222:dbl[])
              n236 = Build Array(w212, w227, w210, w175) -> (w226:dbl[])
              n237 = Build Array(w206, w220, w204, w174) -> (w219:dbl[])
              n238 = Build Array(w203, w217, w201, w216) -> (w215:dbl[])
              n239 = call "ReducedBWSendToNT.vim"("Value In"=w197, "NT Name"="Swerve_Output_Loop_Time" ("Name")) -> ()  [unwired: 1 out]
              n240 = call "ReducedBWSendToNT.vim"("Value In"=w189, "NT Name"="Wrist_Position (deg)") -> ()  [unwired: 1 out]
              n241 = call "ReducedBWSendToNT.vim"("Value In"=w188, "NT Name"="Wrist_Temp (C)") -> ()  [unwired: 1 out]
              n242 = call "ReducedBWSendToNT.vim"("Value In"=w213, "NT Name"="Current_Driver_Profile_Setpoints" ("Name")) -> ()  [unwired: 1 out]
              n243 = call "ReducedBWSendToNT.vim"("Value In"=w231, "NT Name"="Control_Loop_Time" ("Name")) -> ()  [unwired: 1 out]
              n244 = call "ReducedBWSendToNT.vim"("Value In"=w229, "NT Name"="Pose_Loop_Time" ("Name")) -> ()  [unwired: 1 out]
              n245 = call "ReducedBWSendToNT.vim"("Value In"=w193, "NT Name"="Shooter_Speeds (rpm)") -> ()  [unwired: 1 out]
              n246 = call "ReducedBWSendToNT.vim"("Value In"=w192, "NT Name"="Shooter_Temps (C)") -> ()  [unwired: 1 out]
              n247 = call "ReducedBWSendToNT.vim"("Value In"=w169, "NT Name"="Selected_Shooter_Wrist_Angle") -> ()  [unwired: 1 out]
              n248 = call "ReducedBWSendToNT.vim"("Value In"=w173, "NT Name"="Selected_Shooter_Speed") -> ()  [unwired: 1 out]
              n249 = call "ReducedBWSendToNT.vim"("Value In"=w170, "NT Name"="Selected_Shooter_Ratio") -> ()  [unwired: 1 out]
              n250 = call "ReducedBWSendToNT.vim"("Value In"=w179, "NT Name"="Elevator_Goal (in)") -> ()  [unwired: 1 out]
              n251 = call "ReducedBWSendToNT.vim"("Value In"=w176, "NT Name"="Wrist_Goal (deg)") -> ()  [unwired: 1 out]
              n252 = call "ReducedBWSendToNT.vim"("Value In"=w181, "NT Name"="Elevator_Position (in)") -> ()  [unwired: 1 out]
              n253 = call "ReducedBWSendToNT.vim"("Value In"=w180, "NT Name"="Elevator_Temp (C)") -> ()  [unwired: 1 out]
              n254 = call "ReducedBWSendToNT.vim"("Value In"=w165, "NT Name"="Indexer_Temp (C)") -> ()  [unwired: 1 out]
              n255 = call "ReducedBWSendToNT.vim"("Value In"=w162, "NT Name"="Indexer_Speed (rpm)") -> ()  [unwired: 1 out]
              n256 = call "ReducedBWSendToNT.vim"("Value In"=w222, "NT Name"="Swerve_1_Details") -> ()  [unwired: 1 out]
              n257 = call "ReducedBWSendToNT.vim"("Value In"=w226, "NT Name"="Swerve_0_Details") -> ()  [unwired: 1 out]
              n258 = call "ReducedBWSendToNT.vim"("Value In"=w219, "NT Name"="Swerve_2_Details") -> ()  [unwired: 1 out]
              n259 = call "ReducedBWSendToNT.vim"("Value In"=w215, "NT Name"="Swerve_3_Details") -> ()  [unwired: 1 out]
            }
          }
        }
      }
    }
  }
